vi "Read Waveform Channel(Multiple).vi"(7 "Timeout":i32=5000, 8 "error in (no error)":errorcluster, 10 "Number of Reads":i32, 11 "Waveform Paths in":string[](array[string])) -> (0 "error out":errorcluster, 2 "Waveform Data":waveform(dbl)[](array[waveform]), 3 "Waveform Paths out":string[](array[string]))   [LabVIEW 2023, in "FPGA Addon DMA Channels Interleaved System Tests.lvclass"]
uses:
  FPGA Addon DMA Channels Interleaved System Tests.lvclass
  <vilib>/NI VeriStand/Execution/WaveformStreaming/NI_VS Waveform Streaming Interface.lvlib
  <vilib>/NI VeriStand/Execution/WaveformStreaming/Unregister for Waveform Data Events (DBL).vi
  <vilib>/NI VeriStand/Execution/WaveformStreaming/Set Rate for Waveform Stream (Acquisition Rate).vi
  <vilib>/NI VeriStand/Execution/WaveformStreaming/Set Condition for Waveform Stream (All Data).vi
  <vilib>/NI VeriStand/Execution/WaveformStreaming/Register for Waveform Data Events (DBL).vi
  <userlib>/_OpenG.lib/string/string.llb/openg_string.lvlib
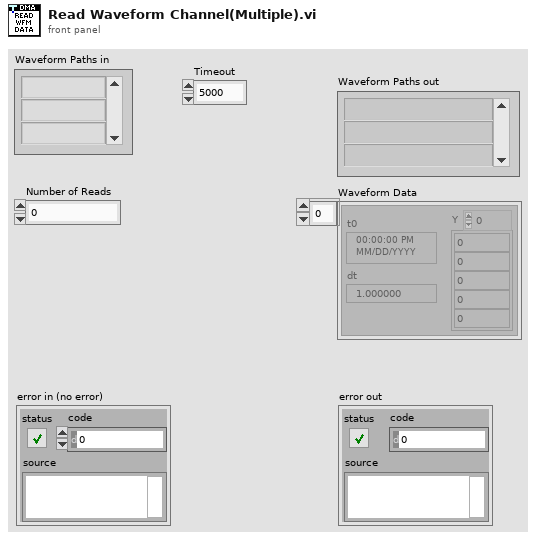
[diagram p1: front panel]
types:
  T1 = typedef "NI_VS Waveform Streaming Interface.lvlib/WaveformStreamSpecification.ctl" = refnum<k24>
  T2 = typedef "NI_VS Waveform Streaming Interface.lvlib/WaveformStreamingAPI.ctl" = refnum<k24>
  T3 = typedef "NI_VS Waveform Streaming Interface.lvlib/Registered Waveform Streams Data Event Refnum (DBL).ctl" = cluster{"Callback Refnum":refnum<k27>, "Data Event":refnum<user-event>, "Event Refnum":refnum<event-registration>, "WaveformDataWatcherDBL":T4}
  T4 = typedef "NI_VS Waveform Streaming Interface.lvlib/WaveformDataWatcherDBL.ctl" = refnum<k24>
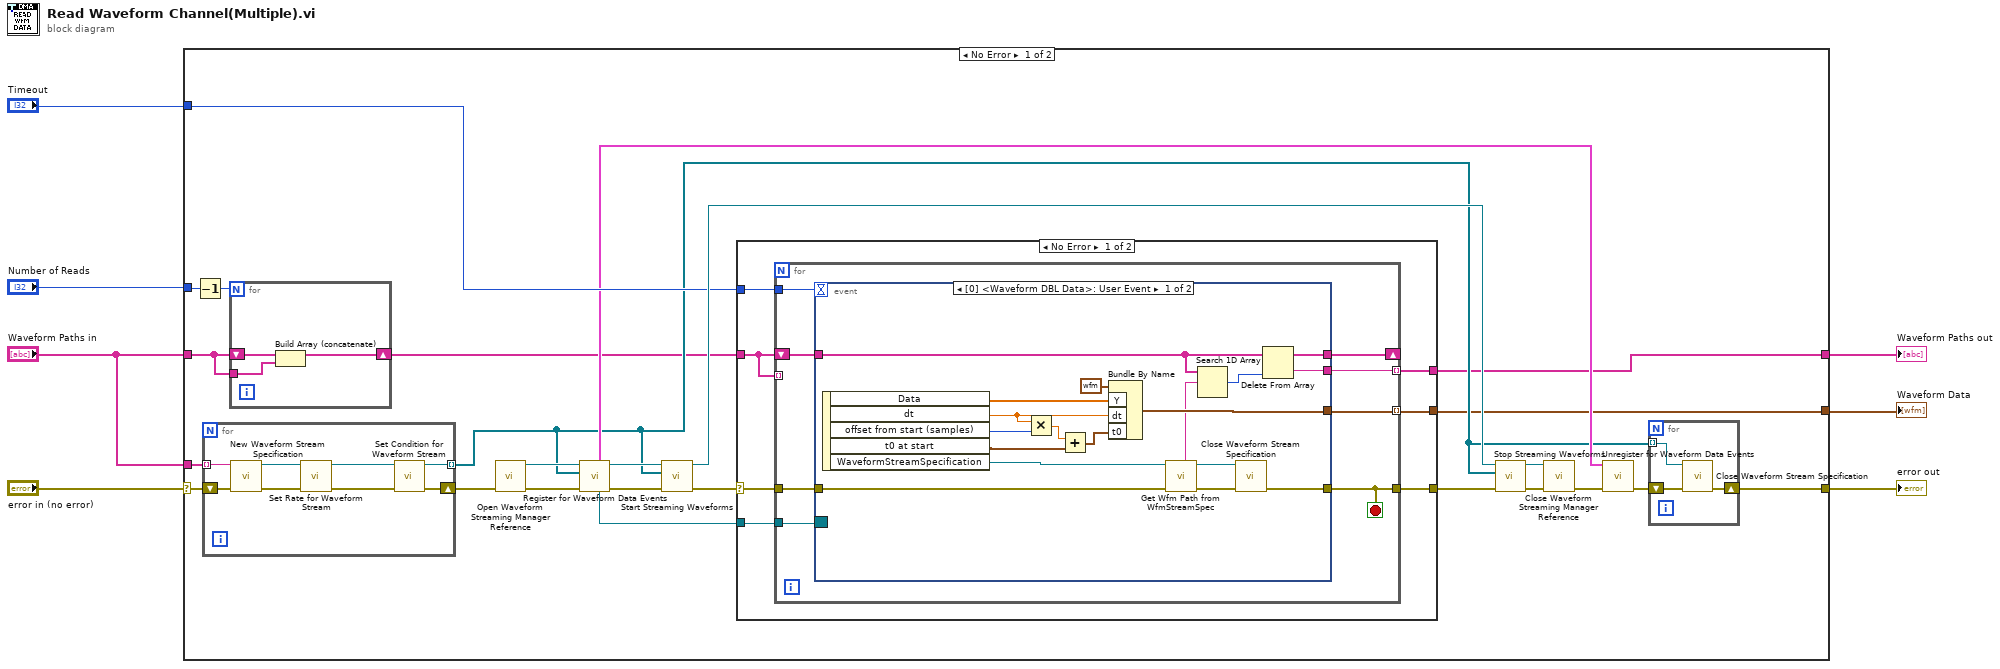
[diagram p0: block diagram]
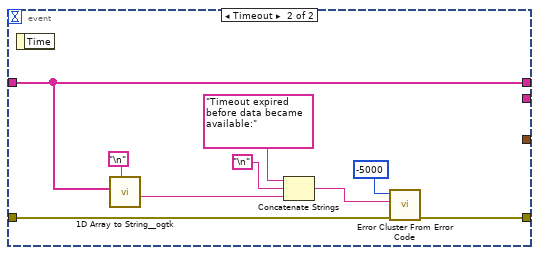
[diagram p2: hidden frame]
diagram:
  n1 = case shown="No Error" "error in (no error)" {
    selector: "error in (no error)" -> [w18 w91]
    tunnel: [w32 w91] -> w7
    tunnel: "Timeout" -> [w17 _]
    tunnel: "Waveform Paths in" -> [w15 _]
    tunnel: "Waveform Paths in" -> [w11 w90]
    tunnel: [w13 _] -> w3
    tunnel: [w12 w90] -> w2
    tunnel: "Number of Reads" -> [w10 _]
    frame No Error {
      n2 = Decrement(x=w10) -> (x-1=w9:i32)
      n3 = for {
        shift-right: [w43] -> w31
        shift-left: w18 -> [w38]
        tunnel: w15 -> [w37] mode=indexing
        tunnel: [w36] -> w14 mode=indexing
        n4 = call <vilib>:"New Waveform Stream Specification.vi"("error in (no error)"=w38, "waveform path"=w37) -> ("error out"=w39:errorcluster, "WaveformStreamSpecification"=w40:T1)  [unwired: 8 in]
        n5 = call-poly <vilib>:"Set Rate for Waveform Stream.vi"("error in (no error)"=w39, "WaveformStreamSpecification in"=w40) -> ("error out"=w41:errorcluster, "WaveformStreamSpecification out"=w42:T1)  [unwired: 8 in]
        n6 = call-poly <vilib>:"Set Condition for Waveform Stream.vi"("error in (no error)"=w41, "WaveformStreamSpecification in"=w42) -> ("error out"=w43:errorcluster, "WaveformStreamSpecification out"=w36:T1)  [unwired: 8 in]
      }
      n7 = for {
        N: w9 -> [_]
        shift-right: [w33] -> w8
        shift-left: w11 -> [w35]
        tunnel: w11 -> [w34]
        n8 = Build Array (concatenate)(w35, w34) -> (w33:string[])
      }
      n9 = call <vilib>:"Open Waveform Streaming Manager Reference.vi"("error in (no error)"=w31) -> ("error out"=w19:errorcluster, "WaveformStreaming"=w20:T2)  [unwired: 9 in]
      n10 = call-poly <vilib>:"Register for Waveform Data Events.vi"("error in (no error)"=w19, "WaveformStreamSpecifications"=w14, "WaveformStreaming in"=w20) -> ("error out"=w21:errorcluster, "WaveformStreaming out"=w22:T2, "waveform data event registration (DBL)"=w24:refnum<event-registration>, "registered waveform data event (DBL)"=w16:T3)  [unwired: 5 in]
      n11 = call <vilib>:"Start Streaming Waveforms.vi"("error in (no error)"=w21, "WaveformStreamSpecifications"=w14, "WaveformStreaming in"=w22) -> ("error out"=w23:errorcluster, "WaveformStreaming out"=w30:T2)  [unwired: 7 in]
      n12 = case shown="No Error" w23 {
        selector: w23 -> [w53 w89]
        tunnel: [w52 w89] -> w25
        tunnel: w24 -> [w51 _]
        tunnel: w17 -> [w50 _]
        tunnel: w8 -> [w49 _]
        tunnel: [w48 _] -> w12
        tunnel: [w47 _] -> w13
        frame No Error {
          n13 = for {
            tunnel: w53 -> [w61]
            tunnel: [w55] -> w52
            tunnel: w51 -> [w60]
            tunnel: w50 -> [w59]
            shift-right: [w57] -> _
            shift-left: w49 -> [w58]
            tunnel: w49 -> [_] mode=indexing
            tunnel: [w56] -> w48 mode=indexing
            tunnel: [w54] -> w47 mode=indexing
            stop <- w55 stop-if-true
            n14 = event shown="[0] <Waveform DBL Data>: User Event" {
              selector: w60 -> [_ _]
              dyn-events: _ -> [_ _]
              timeout: w59 -> [_ _]
              tunnel: w61 -> [w70 w88]
              tunnel: [w73 w87] -> w55
              tunnel: w58 -> [w68 w80]
              tunnel: [w66 w80] -> w57
              tunnel: [w64 _] -> w56
              tunnel: [w63 _] -> w54
              event User Event {
                n15 = event-data() -> ("Data"=w72:dbl[], "dt"=w78:dbl, "offset from start (samples)"=w77:u64, "t0 at start"=w75:timestamp, "WaveformStreamSpecification"=w71:T1)  [unwired: 1 in]
                n16 = Multiply(x=w78, y=w77) -> (x*y=w76:dbl)
                n17 = Add(x=w76, y=w75) -> (x+y=w74:timestamp)
                n18 = Bundle By Name(cluster=waveform(dbl) {"t0"=timestamp(0 s since 1904-01-01), "dt"=1.0, "Y"=[]} ("waveform"), "Y"=w72, "dt"=w78, "t0"=w74) -> (w63:waveform(dbl))
                n19 = call "Get Wfm Path from WfmStreamSpec.vi"("error in (no error)"=w70, ".NET Refnum in"=w71) -> ("error out"=w69:errorcluster, ".NET Refnum out"=w65:T1, "WaveformPath (Duplicate)"=w62:string)  [unwired: 6 in, 1 out]
                n20 = Search 1D Array(1D array=w68, element=w62) -> (index of element=w67:i32)  [unwired: 1 in]
                n21 = call <vilib>:"Close Waveform Stream Specification.vi"("error in (no error)"=w69, "WaveformStreamSpecification"=w65) -> ("error out"=w73:errorcluster)  [unwired: 9 in]
                n22 = Delete From Array(array=w68, index=w67) -> (deleted portion=w64:string, array with subset deleted=w66:string[])  [unwired: 1 in]
              }
              event Timeout {
                n23 = event-data() -> ()  [unwired: 1 in, 1 out]
                n24 = call <userlib>:"1D Array to String__ogtk.vi"("delimiter (Tab)"="\n", "Array of Strings"=w80) -> ("delimited string"=w81:string)  [unwired: 9 in]
                n25 = Concatenate Strings("Timeout expired before data became available:" ("error message (\"\")"), "\n", w81) -> (w83:string)
                n26 = call <vilib>:"Error Cluster From Error Code.vi"("error in (no error)"=w88, "error message (\"\")"=w83, "error code (0)"=-5000) -> ("error out"=w87:errorcluster)  [unwired: 6 in]
              }
            }
          }
        }
        frame Error {
        }
      }
      n27 = call <vilib>:"Stop Streaming Waveforms.vi"("error in (no error)"=w25, "WaveformStreamSpecifications"=w14, "WaveformStreaming in"=w30) -> ("error out"=w26:errorcluster, "WaveformStreaming out"=w27:T2)  [unwired: 7 in]
      n28 = call <vilib>:"Close Waveform Streaming Manager Reference.vi"("error in (no error)"=w26, "WaveformStreaming"=w27) -> ("error out"=w28:errorcluster)  [unwired: 9 in]
      n29 = call-poly <vilib>:"Unregister for Waveform Data Events.vi"("error in (no error)"=w28, "registered waveform data event (DBL)"=w16) -> ("error out"=w29:errorcluster)  [unwired: 9 in]
      n30 = for {
        shift-right: [w45] -> w32
        shift-left: w29 -> [w46]
        tunnel: w14 -> [w44] mode=indexing
        n31 = call <vilib>:"Close Waveform Stream Specification.vi"("error in (no error)"=w46, "WaveformStreamSpecification"=w44) -> ("error out"=w45:errorcluster)  [unwired: 9 in]
      }
    }
    frame Error {
    }
  }
  "error out" <- w7
  "Waveform Paths out" <- w2
  "Waveform Data" <- w3
